vi "Acquisition_a.vi"() -> (4 "Acquired_Data":dbl(graph))   [LabVIEW 2021]
doc: "This VI acquire data that were generated be the Generator VI.\nTransfer of thet data happens under Global variable."
uses:
  Global_Variables/Generate_Data_Global.vi
panel:
  out "Error_Out":errorcluster
  in  "Error_In":errorcluster
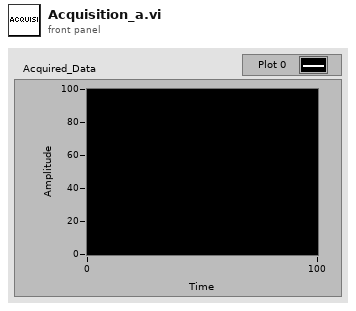
[diagram p1: front panel]
types:
  T1 = enum16{"Left Button", "Center Button", "Right Button", "Window Close"}
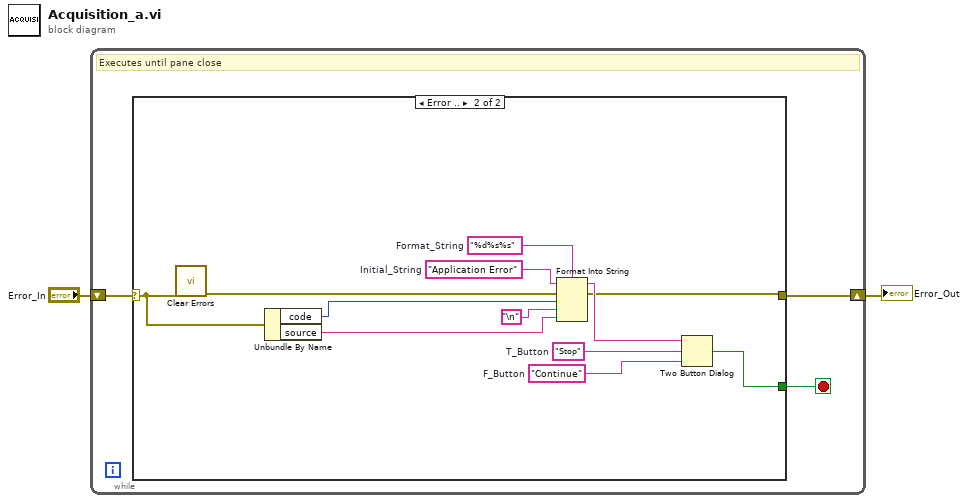
[diagram p0: block diagram]
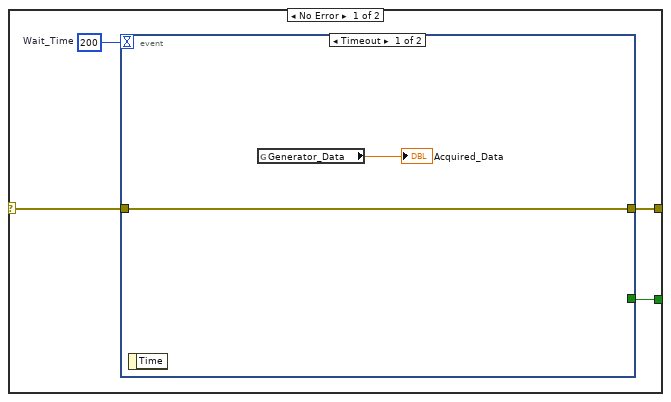
[diagram p2: hidden frame]
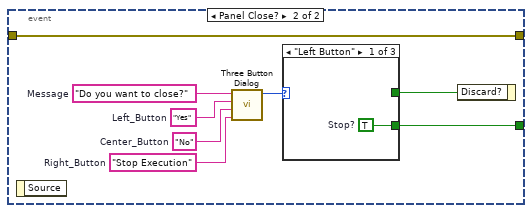
[diagram p3: hidden frame]
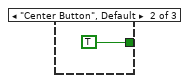
[diagram p4: hidden frame]
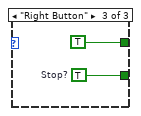
[diagram p5: hidden frame]
diagram:
  n1 = while {
    shift-right: [w3] -> w1
    shift-left: "Error_In" -> [w4]
    stop <- w5 stop-if-true
    # "Executes until pane close"
    n2 = case shown="Error .." w4 {
      selector: w4 -> [w6 w29]
      tunnel: [w8 w24] -> w5
      tunnel: [w7 w27] -> w3
      frame No Error {
        w9 = 200  # Wait_Time
        n3 = event shown="[0] Timeout" {
          selector: _ -> [_ _]
          dyn-events: _ -> [_ _]
          timeout: w9 -> [_ _]
          tunnel: [_ w13] -> w8
          tunnel: [w10 w12] -> w7
          tunnel: w6 -> [w10 w12]
          event Timeout {
            n4 = event-data() -> ()  [unwired: 1 in, 1 out]
            n5 = global read "Generate_Data_Global.vi" "Generator_Data"() -> (→"Acquired_Data":dbl)
          }
          event Panel Close? {
            w16 = "Stop Execution"  # Right_Button
            w17 = "No"  # Center_Button
            w18 = "Yes"  # Left_Button
            w19 = "Do you want to close?"  # Message
            n6 = event-data() -> ()  [unwired: 1 in, 1 out]
            n7 = call <vilib>:"Three Button Dialog.vi"("Right Button Text (\"Cancel\")"=w16, "Center Button Text (\"No\")"=w17, "Left Button Text (\"Yes\")"=w18, "message"=w19) -> ("Which Button?"=w15:T1)  [unwired: 7 in]
            n8 = case shown="\"Left Button\"" w15 {
              tunnel: [_ TRUE ("Discard?") TRUE ("Discard?")] -> w14
              tunnel: [w20 _ w23] -> w13
              frame "Left Button" {
                w20 = TRUE  # Stop?
              }
              frame "Center Button", Default {
              }
              frame "Right Button" {
                w23 = TRUE  # Stop?
              }
            }
            n9 = event-data("Discard?"=w14) -> ()  [unwired: 1 in, 1 out]
          }
        }
      }
      frame Error {
        w31 = "%d%s%s"  # Format_String
        w32 = "Application Error"  # Initial_String
        w33 = "Stop"  # T_Button
        w34 = "Continue"  # F_Button
        n10 = call <vilib>:"Clear Errors.vi"("error in (no error)"=w29) -> ("error out"=w28:errorcluster)  [unwired: 5 in, 1 out]
        n11 = Unbundle By Name(w29) -> ("code"=w25:i32, "source"=w26:string)
        n12 = Format Into String(format string=w31, initial string=w32, error in=w28, w25, "\n", w26) -> (resulting string=w35:string, error out=w27:errorcluster)
        n13 = Two Button Dialog(message=w35, 1:w34, 2:w33) -> (T button?=w24:bool)
      }
    }
  }
  "Error_Out" <- w1
